vi "Initialization VI.vi"(8 "error in (no error)":errorcluster, 10 "Custom XML":string, 11 "Device Item Ref in":T1 format="%.0x") -> (0 "error out":errorcluster, 3 "Device Item Ref out":T1 format="%.0x")   [LabVIEW 2015, in "Host Heartbeat System Explorer.lvlib"]
uses:
  Host Heartbeat System Explorer.lvlib
  <vilib>/NI Veristand/Custom Device API/Custom Device Item Ref.ctl
  <vilib>/NI Veristand/Custom Device API/Custom Device Channel.ctl
  <vilib>/NI Veristand/Custom Device API/Custom Device Channel Type.ctl
  <vilib>/NI Veristand/Custom Device API/Custom Device API.lvlib
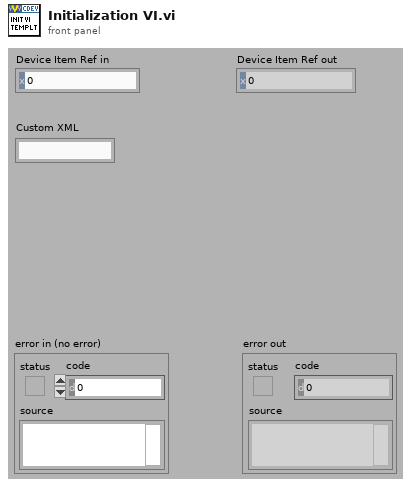
[diagram p1: front panel]
types:
  T1 = typedef "Custom Device API.lvlib/Custom Device Item Ref.ctl" = u64
  T2 = typedef "Custom Device API.lvlib/Custom Device Channel.ctl" = cluster{"Type":T3, "Units":string, "Default Value":dbl, "Faultable":bool, "Scalable":bool}
  T3 = typedef "Custom Device API.lvlib/Custom Device Channel Type.ctl" = enum16{"Input", "Output"}
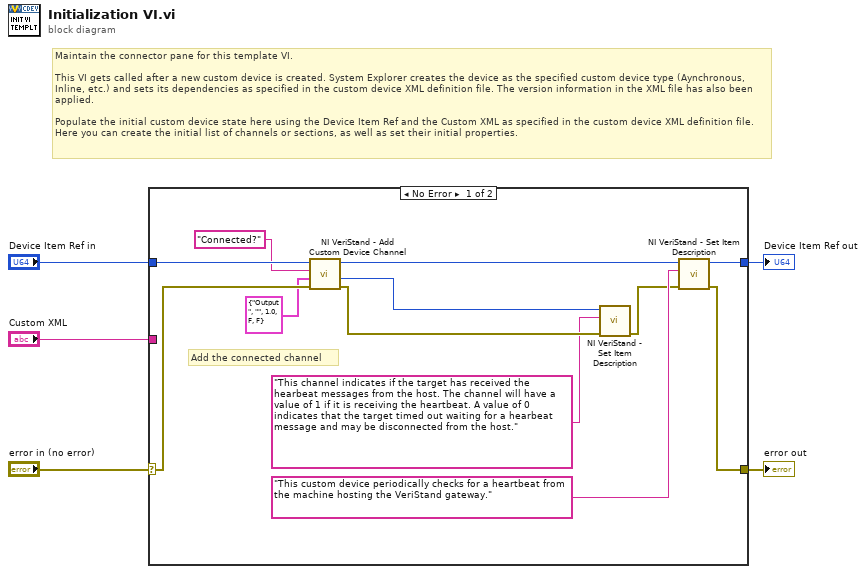
[diagram p0: block diagram]
diagram:
  # "Maintain the connector pane for this template VI.\n\nThis VI gets called after a new custom device is created. System Explorer creates the device as the specified custom device type (Aynchronous, Inline, etc.) and sets its dependencies as specified in the custom device XML definition file. The version information in the XML file has also been applied.\n\nPopulate the initial custom device state here using the Device Item Ref and the Custom XML as specified in the custom device XML definition file. Here you can create the initial list of channels or sections, as well as set their initial properties."
  n1 = case shown="No Error" "error in (no error)" {
    selector: "error in (no error)" -> [w16 w19]
    tunnel: [w12 w19] -> w5
    tunnel: [w11 w18] -> w3
    tunnel: "Device Item Ref in" -> [w17 w18]
    tunnel: "Custom XML" -> [_ _]
    frame No Error {
      # "Add the connected channel"
      n2 = call <vilib>:"NI VeriStand - Add Custom Device Channel.vi"("error in (no error)"=w16, "Channel"=T2 {"Type"=enum."Output", "Units"="", "Default Value"=1.0, "Faultable"=FALSE, "Scalable"=FALSE}, "Channel Name"="Connected?", "Parent Ref in"=w17) -> ("error out"=w9:errorcluster, "Channel Ref"=w8:T1, "Parent Ref out"=w13:T1)  [unwired: 4 in, 1 out]
      n3 = call <vilib>:"NI VeriStand - Set Item Description.vi"("error in (no error)"=w9, "Description"="This channel indicates if the target has received the hearbeat messages from the host. The channel will have a value of 1 if it is receiving the heartbeat. A value of 0 indicates that the target timed out waiting for a hearbeat message and may be disconnected from the host.", "Item Ref in"=w8) -> ("error out"=w7:errorcluster)  [unwired: 6 in, 2 out]
      n4 = call <vilib>:"NI VeriStand - Set Item Description.vi"("error in (no error)"=w7, "Description"="This custom device periodically checks for a heartbeat from the machine hosting the VeriStand gateway.", "Item Ref in"=w13) -> ("error out"=w12:errorcluster, "Item Ref out"=w11:T1)  [unwired: 6 in, 1 out]
    }
    frame Error {
    }
  }
  "error out" <- w5
  "Device Item Ref out" <- w3
